vi "set_ref_clus_RootsPumpLCW.vi"(6 "variable_reference":T1, 10 "array_flow":dbl[](array[numeric]), 11 "status":bool) -> ()   [LabVIEW 2019]
uses:
  cluster_ref_RootsPumpLCW.ctl
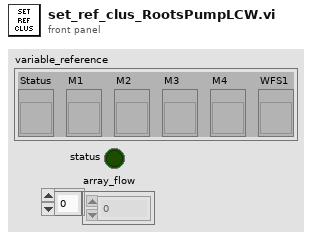
[diagram p1: front panel]
types:
  T1 = typedef "cluster_ref_RootsPumpLCW.ctl" = cluster{"Status":refnum<vi>, "M1":refnum<vi>, "M2":refnum<vi>, "M3":refnum<vi>, "M4":refnum<vi>, "WFS1":refnum<vi>}
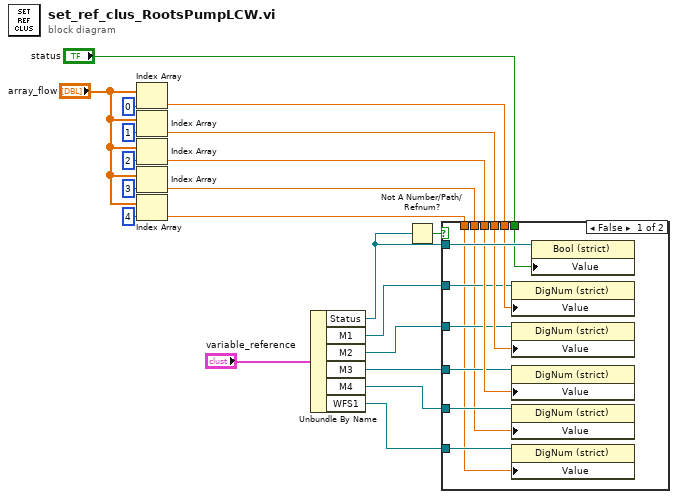
[diagram p0: block diagram]
diagram:
  n1 = Index Array(array="array_flow", index=0) -> (element=w11:dbl)
  n2 = Index Array(array="array_flow", index=1) -> (element=w4:dbl)
  n3 = Index Array(array="array_flow", index=2) -> (element=w3:dbl)
  n4 = Index Array(array="array_flow", index=3) -> (element=w2:dbl)
  n5 = Index Array(array="array_flow", index=4) -> (element=w1:dbl)
  n6 = Unbundle By Name("variable_reference") -> ("Status"=w16:refnum<vi>, "M1"=w17:refnum<vi>, "M2"=w18:refnum<vi>, "M3"=w19:refnum<vi>, "M4"=w13:refnum<vi>, "WFS1"=w12:refnum<vi>)
  n7 = Not A Number/Path/Refnum?(number/path/refnum=w16) -> (NaN/Path/Refnum?=w20:bool)
  n8 = case shown="False" w20 {
    tunnel: w11 -> [w27 _]
    tunnel: w4 -> [w29 _]
    tunnel: w3 -> [w30 _]
    tunnel: w17 -> [w25 _]
    tunnel: w18 -> [w28 _]
    tunnel: w19 -> [w26 _]
    tunnel: w16 -> [w32 _]
    tunnel: "status" -> [w31 _]
    tunnel: w13 -> [w24 _]
    tunnel: w12 -> [w23 _]
    tunnel: w2 -> [w22 _]
    tunnel: w1 -> [w21 _]
    frame False {
      n9 = property class="DigNum (strict)"(reference=w25, "Value"=w27) -> ()  [unwired: 1 in, 2 out]
      n10 = property class="DigNum (strict)"(reference=w28, "Value"=w29) -> ()  [unwired: 1 in, 2 out]
      n11 = property class="DigNum (strict)"(reference=w26, "Value"=w30) -> ()  [unwired: 1 in, 2 out]
      n12 = property class="DigNum (strict)"(reference=w24, "Value"=w22) -> ()  [unwired: 1 in, 2 out]
      n13 = property class="DigNum (strict)"(reference=w23, "Value"=w21) -> ()  [unwired: 1 in, 2 out]
      n14 = property class="Bool (strict)"(reference=w32, "Value"=w31) -> ()  [unwired: 1 in, 2 out]
    }
    frame True {
    }
  }
